vi "Thermometers.vi"() -> ()   [LabVIEW 2023]
panel:
  out "Thermometers":cluster{"T_H":dbl, "T_C1":dbl, "T_C2":dbl}
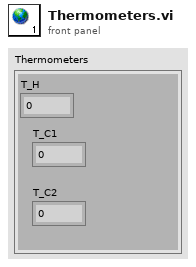
[diagram p1: front panel]
diagram:
